vi "ConfigSQLiteSettingDialog.vi"() -> ()   [LabVIEW 2018]
doc: "[Ver 1.00]\nDESCRIPTION\nThis is is the user interface for the config ini data. This can be used as a pattern to apply to all programs to ensure detail is kept out of the code.\n\nERROR HANDLING\nThrow, log error\n\n------------------------------------------------------------------------\n[Ver 1.00]\nSWatts SSDC 07/04/03"
uses:
  System Config Data Manager Parameter.ctl
  Datamanager.ctl
  <vilib>/event_ctls.llb/eventsource.ctl
  ConfigScreen States.ctl
  ConfigCommand.ctl
  Database/SystemdBCommands.ctl
  Error/ErrorCommand.ctl
  StoreCommand.ctl
  <vilib>/Utility/NIReport.llb/NI_report.lvclass
panel:
  in  "Source":T1 items=["LabVIEW UI"=0, "ActiveX"=1, "User Event"=25]
  in  "Save As Button":bool
  in  "Lock Button":bool
  in  "Section":T2
  in  "Table Control":string[][](table)=[["Password"], ["PhysicsLIMs"], ["LIMSSASDBF"], ["a4bld"], ["User"], ["RUN"], ["N:\\LIMS\\Reports\\"], ["C:\\AWE\\Physics LIMS\\HelpFiles\\Help.html"], ["C:\\AWE\\Physics LIMS\\HelpFiles\\PASStaff.html"], ["C:\\AWE\\Physics LIMS\\HelpFiles\\SASWAS.html"], ["C:\\AWE\\Physics LIMS\\HelpFiles\\PASRoutine.html"], ["C:\\AWE\\Physics LIMS\\HelpFiles\\BeHelp.html"], ["C:\\AWE\\Physics LIMS\\HelpFiles\\Building.html"], ["C:\\AWE\\Physics LIMS\\HelpFiles\\PASVisitor.html"], ["C:\\AWE\\Physics LIMS\\HelpFiles\\BeScheduled.html"], ["C:\\AWE\\Physics LIMS\\HelpFiles\\BeUnscheduled.html"], ["C:\\AWE\\Physics LIMS\\HelpFiles\\BeReports.html"], ["C:\\AWE\\Physics LIMS\\HelpFiles\\PASReports.html"], ["C:\\AWE\\Physics LIMS\\HelpFiles\\QA.html"], ["C:\\AWE\\Physics LIMS\\HelpFiles\\Browse.html"], ["C:\\AWE\\Physics LIMS\\HelpFiles\\LEAD.html"], ["C:\\PHYSICSLIMSRB\\"], ["C:/PHYSICSLIMSRB/"], ["C:\\Program Files\\Seagull\\BarTender\\8.0\\BarTend.exe"], ["C:\\AWE\\Physics LIMS\\Documents\\BartenderLabels\\"], ["10"], [""], [""], [""], [""], [""], [""], [""], [""], [""], [""], [""], [""], [""], [""], [""], [""], [""], [""], [""], [""], [""], [""], [""], [""], ["MANUAL VIS PAS RA.btw"], [""], [""], [""], [""], [""], ["A:\\"], ["N:\\LIMS\\IPSIS\\"], ["C:\\AWE\\Physics LIMS\\Documents\\BartenderLabels\\BEWorklist.btw"], ["N:\\LIMS\\BEFILES\\"], ["COM11"], ["0.02001|0.10|0.50|1.0|2.0"], [">0.02<0.1|>=0.1<0.5|>=0.5<1|>=1<2|>=2"], ["0.02001|0.1|0.5|1.0|2.0"], [">0.02<0.1|>=0.1<0.5|>=0.5<1|>=1<2|>=2"], ["C:\\AWE\\Physics LIMS\\Documents\\SAS\\DailyHPR59.btw"], ["SSDCPDF"]]
  in  "SaveButton":bool
  in  "OK":bool
  in  "PrintButton":bool
  in  "SysParameter":T3=enum."RunStatus"
  in  "Version":string(combo)
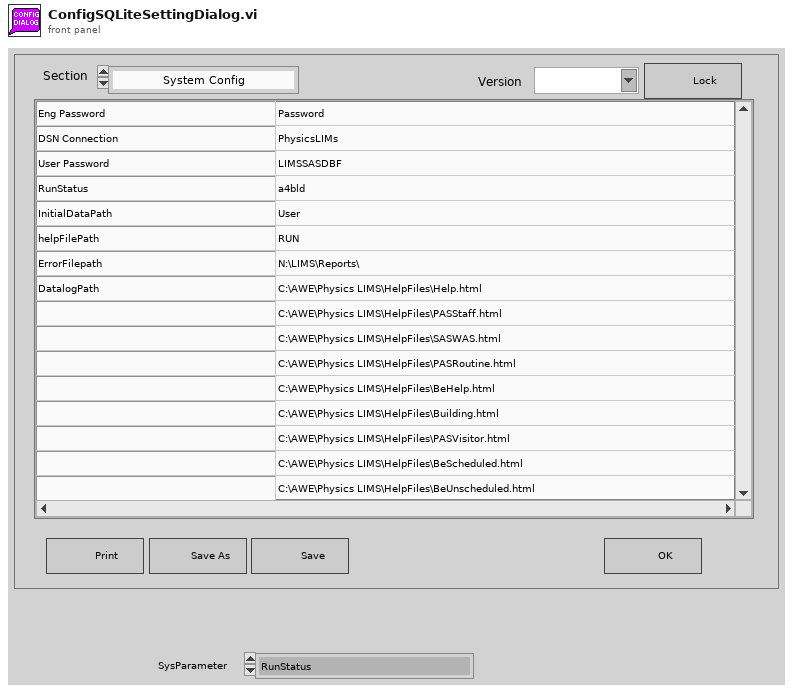
[diagram p1: front panel]
types:
  T1 = typedef "eventsource.ctl" = u32
  T2 = typedef "Datamanager.ctl" = enum16{"System Config"}
  T3 = typedef "System Config Data Manager Parameter.ctl" = enum16{"Eng Password", "DSN Connection", "User Password", "RunStatus", "InitialDataPath", "helpFilePath", "ErrorFilepath", "DatalogPath", "Hello"}
  T4 = typedef "ConfigScreen States.ctl" = enum16{"Initialize", "Run"}
  T5 = typedef "SystemdBCommands.ctl" = enum16{"No Command - Error", "Set Filepath", "Connect dB", "Disconnect dB", "Start Transaction", "Commit", "Rollback", "Describe Table", "Select All From Table", "Fetch Query", "Count Records In Table", "Get User Information", "Get System Config", "Insert New System Config", "UPDATE User Info", "Insert New User", "Get Versions", "Update Key", "Set Version to Default", "Get Default Version", "INSERT Error", "UPDATE Error", "DELETE Errors", "Get All Errors", "Get #Errors for Error"}
  T6 = typedef "ConfigCommand.ctl" = enum16{"No Command - Error", "Initialise Config SQLite", "Save Config", "Get Key", "Set Key", "Update Key", "Get Latest Config Data", "Get Config Data for Version", "Get Default Config Data"}
  T7 = typedef "ErrorCommand.ctl" = enum16{"No Command - Error", "Set to Dev Mode", "Set To Released Mode", "Set Error", "Log Error", "Throw Error", "Log & Throw Error", "Set Error Timed"}
  T8 = typedef "StoreCommand.ctl" = enum16{"No Command - Error", "Store New Version From Inputs", "Update From Input", "Store from dB"}
  T9 = enum16{"Standard Report", "HTML", "Word", "Excel"}
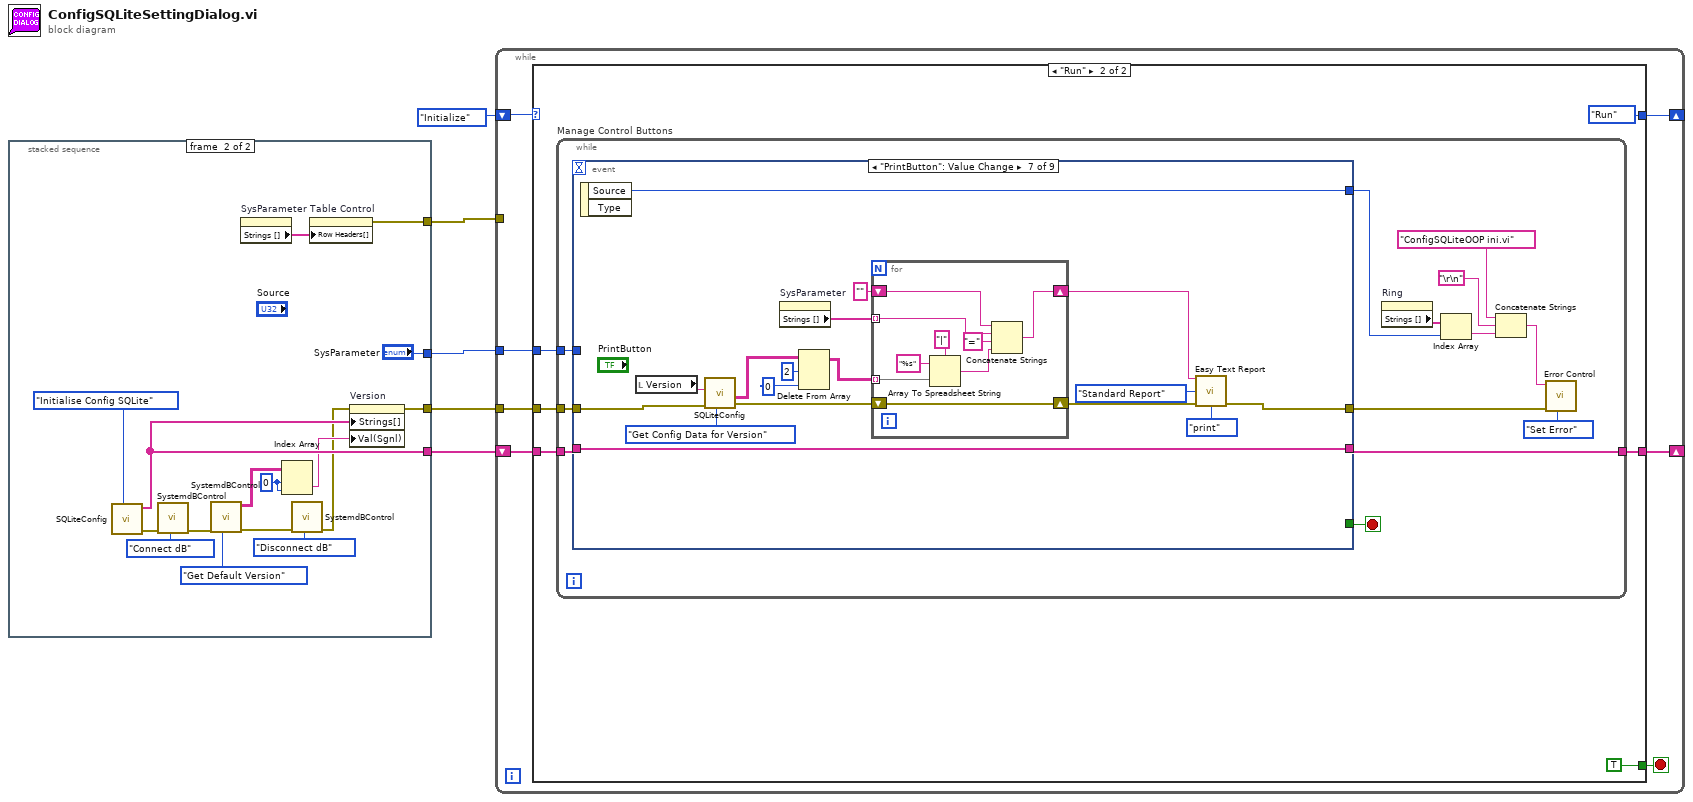
[diagram p0: block diagram]
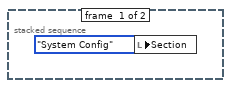
[diagram p2: hidden frame]
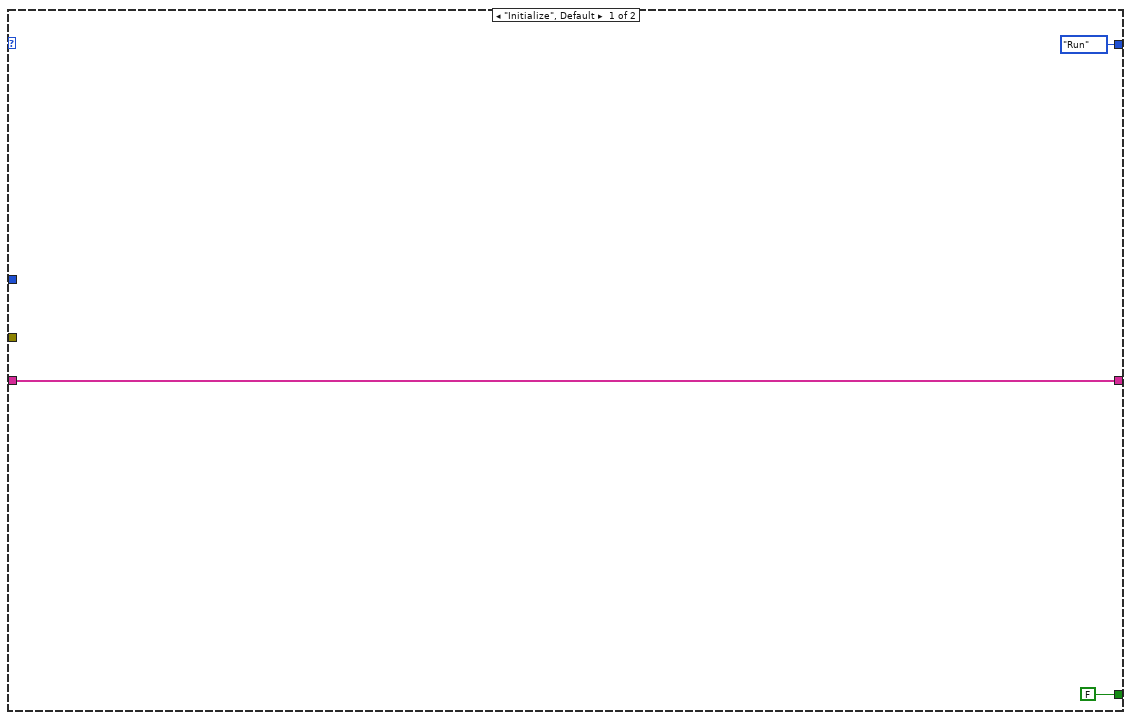
[diagram p3: hidden frame]
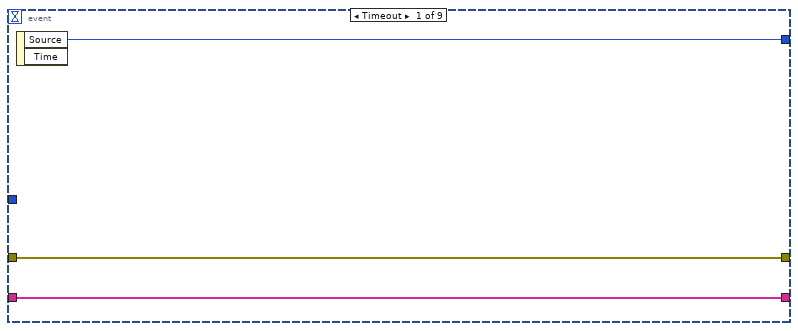
[diagram p4: hidden frame]
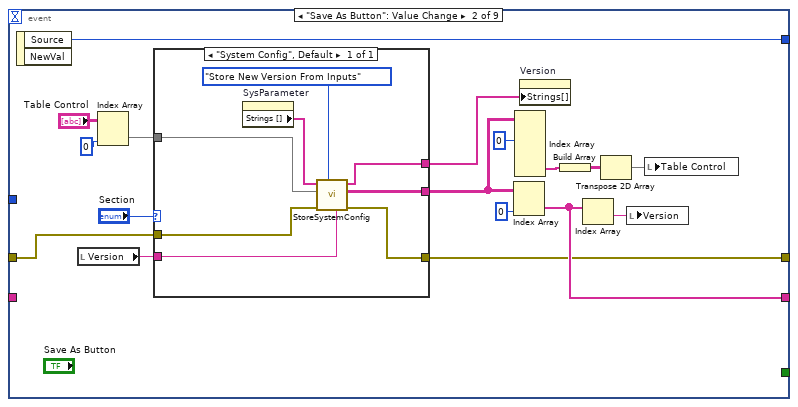
[diagram p5: hidden frame]
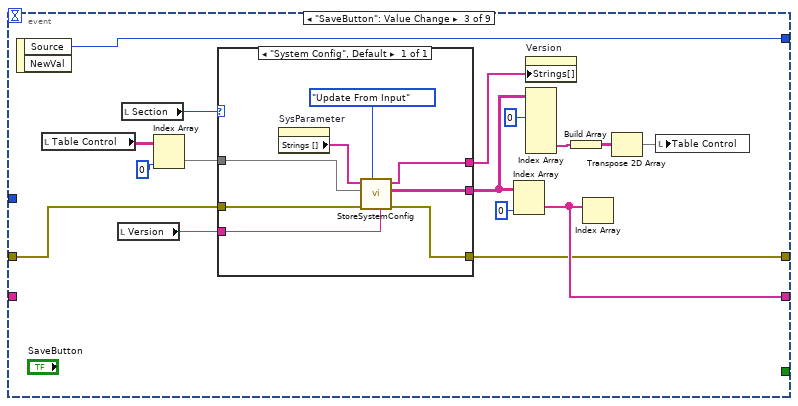
[diagram p6: hidden frame]
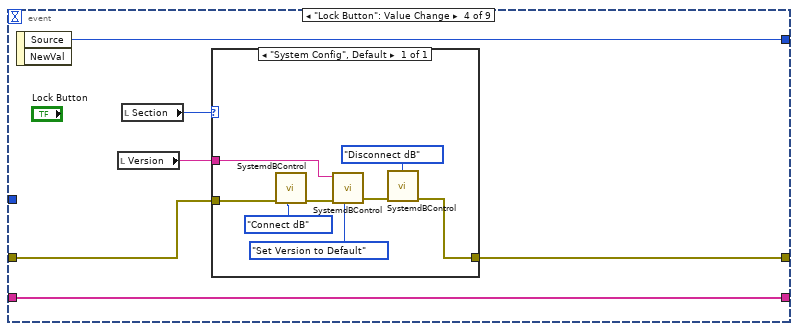
[diagram p7: hidden frame]
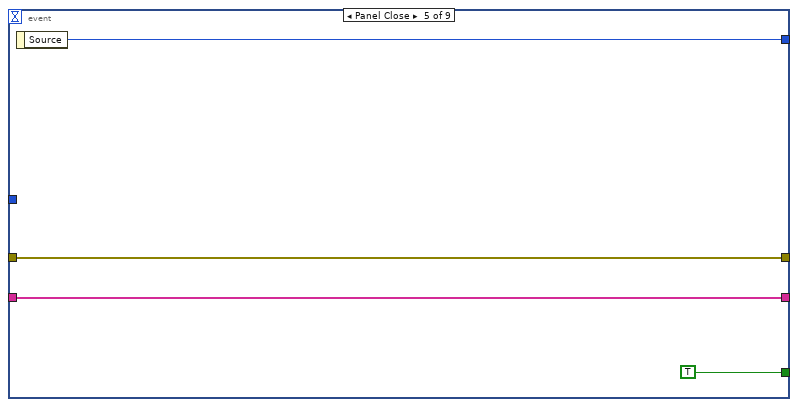
[diagram p8: hidden frame]
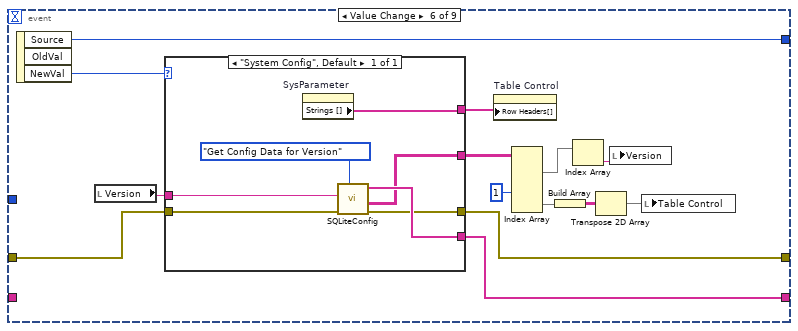
[diagram p9: hidden frame]
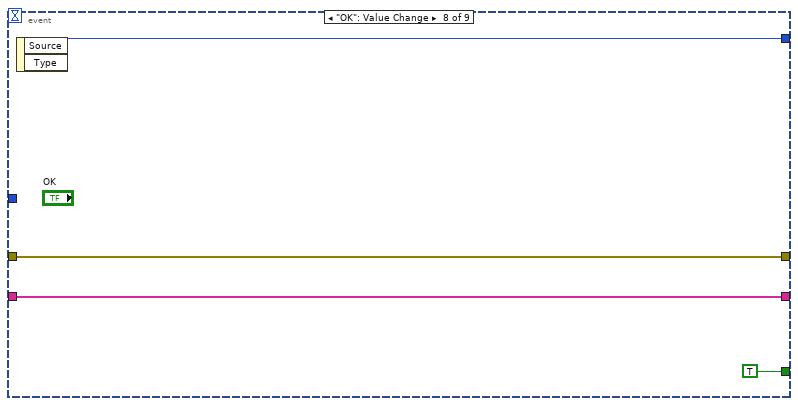
[diagram p10: hidden frame]
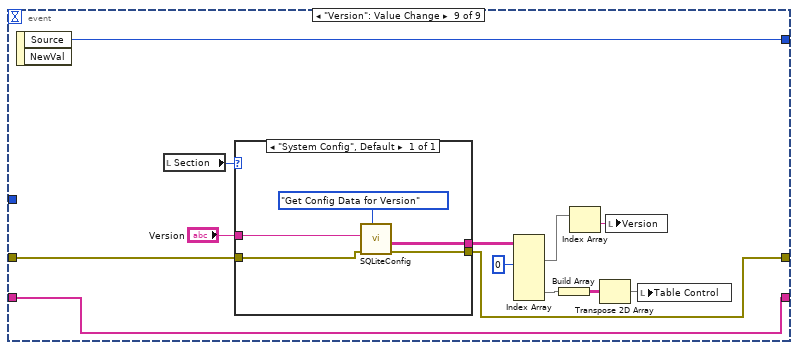
[diagram p11: hidden frame]
diagram:
  n1 = stacked-sequence {
    tunnel: [_ w20] -> w4
    tunnel: [_ "SysParameter"] -> w3
    tunnel: [_ w21] -> w2
    tunnel: [_ w19] -> w1
    frame #0 {
      n2 = local write "Section"(Datamanager."System Config" ("Section")) -> ()
    }
    frame #1 {
      w14 = 0 ("index (row)")
      n3 = call "SQLiteConfig.vi"("ConfigCommand"=ConfigCommand."Initialise Config SQLite") -> ("error out"=w9:errorcluster, "AvailableVersions"=w19:string[])  [unwired: 4 in, 2 out]
      n4 = call "SystemdBControl.vi"("Command"=SystemdBCommands."Connect dB", "error in (no error)"=w9) -> ("error out"=w8:errorcluster)  [unwired: 5 in, 2 out]
      n5 = call "SystemdBControl.vi"("Command"=SystemdBCommands."Get Default Version", "error in (no error)"=w8) -> ("error out"=w11:errorcluster, "Data Out"=w15:string[][])  [unwired: 5 in, 1 out]
      n6 = property on="SysParameter" class="Enum (strict)"() -> ("Strings []"=w18:string[])  [unwired: 2 in, 2 out]
      n7 = Index Array(array=w15, index (row)=w14, index (col)=w14) -> (element=w13:string)
      n8 = call "SystemdBControl.vi"("Command"=SystemdBCommands."Disconnect dB", "error in (no error)"=w11) -> ("error out"=w12:errorcluster)  [unwired: 5 in, 2 out]
      n9 = property on="Table Control" class="Tbl (strict)"("Row Headers[]"=w18) -> (error out=w21:errorcluster)  [unwired: 2 in, 1 out]
      n10 = property on="Version" class="CmbBox"(error in=w12, "Strings[]"=w19, "Val(Sgnl)"=w13) -> (error out=w20:errorcluster)  [unwired: 1 in, 1 out]
    }
  }
  n11 = while {
    shift-right: [w28] -> _
    shift-left: ConfigScreen_States."Initialize" ("Screen State") -> [w29]
    tunnel: w4 -> [w23]
    tunnel: w3 -> [w26]
    tunnel: w2 -> [_]
    shift-right: [w24] -> _
    shift-left: w1 -> [w25]
    stop <- w27 stop-if-true
    n12 = case shown="\"Run\"" w29 {
      tunnel: [ConfigScreen_States."Run" ("Screen State") ConfigScreen_States."Run" ("Screen State")] -> w28
      tunnel: [FALSE TRUE] -> w27
      tunnel: w26 -> [_ w35]
      tunnel: w25 -> [w30 w36]
      tunnel: [w30 w34] -> w24
      tunnel: w23 -> [_ w33]
      frame "Initialize", Default {
      }
      frame "Run" {
        n13 = while "Manage Control Buttons" {
          tunnel: w36 -> [w50]
          tunnel: w35 -> [w49]
          tunnel: [w48] -> w34
          tunnel: w33 -> [w47]
          stop <- w51 stop-if-true
          n14 = event shown="[6] \"PrintButton\": Value Change" {
            selector: _ -> [_ _ _ _ _ _ _ _ _]
            dyn-events: _ -> [_ _ _ _ _ _ _ _ _]
            timeout: _ -> [_ _ _ _ _ _ _ _ _]
            tunnel: [_ _ _ _ TRUE _ _ TRUE _] -> w51
            tunnel: w50 -> [w54 _ _ w107 w120 _ w159 w171 w180]
            tunnel: w49 -> [_ _ _ _ _ _ _ _ _]
            tunnel: [w54 w66 w92 w107 w120 w127 w159 w171 w180] -> w48
            tunnel: w47 -> [w52 w56 w81 w106 w118 w124 w156 w169 w175]
            tunnel: [w52 w55 w80 w104 w118 w123 w149 w169 w174] -> w42
            tunnel: [w53 w57 w82 w105 w119 w122 w148 w170 w173] -> w40
            event Timeout {
              n15 = event-data() -> ("Source"=w53:T1)  [unwired: 1 in, 1 out]
            }
            event "Save As Button": Value Change {
              n16 = event-data() -> ("Source"=w57:T1)  [unwired: 1 in, 1 out]
              n17 = local read "Version"() -> (w58:string)
              n18 = Index Array(array="Table Control", index (col)=0 ("disabled index (col)")) -> (element=w70:string[])  [unwired: 1 in]
              n19 = case shown="\"System Config\", Default" "Section" {
                tunnel: w70 -> [w79]
                tunnel: [w78] -> w60
                tunnel: [w77] -> w62
                tunnel: w58 -> [w74]
                tunnel: w56 -> [w73]
                tunnel: [w72] -> w55
                frame "System Config", Default {
                  n20 = property on="SysParameter" class="Enum (strict)"() -> ("Strings []"=w76:string[])  [unwired: 2 in, 2 out]
                  n21 = call "StoreSystemConfig.vi"("Version"=w74, "StoreConfigCommand"=StoreCommand."Store New Version From Inputs", "error in"=w73, "Table Control"=w79, "Strings []"=w76) -> ("error out"=w72:errorcluster, "All Data"=w78:string[][], "AvailableVersions"=w77:string[])  [unwired: 2 in]
                }
              }
              n22 = Index Array(array=w60, index (col)=0 ("disabled index (col)")) -> (element=w66:string[])  [unwired: 1 in]
              n23 = Index Array(array=w60, index (col) #1=0 ("disabled index (col)")) -> (element #3=w64:string[])  [unwired: 5 in, 2 out]
              n24 = property on="Version" class="CmbBox"("Strings[]"=w62) -> ()  [unwired: 2 in, 2 out]
              n25 = Build Array(w64) -> (w65:string[][])
              n26 = Index Array(array=w66) -> (element=w67:string)  [unwired: 1 in]
              n27 = Transpose 2D Array(2D array=w65) -> (transposed array=w63:string[][])
              n28 = local write "Version"(w67) -> ()
              n29 = local write "Table Control"(w63) -> ()
            }
            event "SaveButton": Value Change {
              n30 = event-data() -> ("Source"=w82:T1)  [unwired: 1 in, 1 out]
              n31 = local read "Table Control"() -> (w84:string[][])
              n32 = local read "Version"() -> (w85:string)
              n33 = local read "Section"() -> (w83:T2)
              n34 = Index Array(array=w84, index (col)=0 ("disabled index (col)")) -> (element=w94:string[])  [unwired: 1 in]
              n35 = case shown="\"System Config\", Default" w83 {
                tunnel: w94 -> [w103]
                tunnel: [w102] -> w87
                tunnel: [w101] -> w88
                tunnel: w85 -> [w98]
                tunnel: w81 -> [w97]
                tunnel: [w96] -> w80
                frame "System Config", Default {
                  n36 = property on="SysParameter" class="Enum (strict)"() -> ("Strings []"=w100:string[])  [unwired: 2 in, 2 out]
                  n37 = call "StoreSystemConfig.vi"("Version"=w98, "StoreConfigCommand"=StoreCommand."Update From Input", "error in"=w97, "Table Control"=w103, "Strings []"=w100) -> ("error out"=w96:errorcluster, "All Data"=w102:string[][], "AvailableVersions"=w101:string[])  [unwired: 2 in]
                }
              }
              n38 = Index Array(array=w87, index (col)=0 ("disabled index (col)")) -> (element=w92:string[])  [unwired: 1 in]
              n39 = property on="Version" class="CmbBox"("Strings[]"=w88) -> ()  [unwired: 2 in, 2 out]
              n40 = Index Array(array=w87, index (col) #1=0 ("disabled index (col)")) -> (element #3=w90:string[])  [unwired: 5 in, 2 out]
              n41 = Build Array(w90) -> (w91:string[][])
              n42 = Index Array(array=w92) -> ()  [unwired: 1 in, 1 out]
              n43 = Transpose 2D Array(2D array=w91) -> (transposed array=w89:string[][])
              n44 = local write "Table Control"(w89) -> ()
            }
            event "Lock Button": Value Change {
              n45 = event-data() -> ("Source"=w105:T1)  [unwired: 1 in, 1 out]
              n46 = local read "Version"() -> (w109:string)
              n47 = local read "Section"() -> (w108:T2)
              n48 = case shown="\"System Config\", Default" w108 {
                tunnel: w109 -> [w112]
                tunnel: w106 -> [w111]
                tunnel: [w110] -> w104
                frame "System Config", Default {
                  n49 = call "SystemdBControl.vi"("Command"=SystemdBCommands."Connect dB", "error in (no error)"=w111) -> ("error out"=w116:errorcluster)  [unwired: 5 in, 2 out]
                  n50 = call "SystemdBControl.vi"("Command"=SystemdBCommands."Set Version to Default", "error in (no error)"=w116, "Data In"=w112) -> ("error out"=w114:errorcluster)  [unwired: 4 in, 2 out]
                  n51 = call "SystemdBControl.vi"("Command"=SystemdBCommands."Disconnect dB", "error in (no error)"=w114) -> ("error out"=w110:errorcluster)  [unwired: 5 in, 2 out]
                }
              }
            }
            event Panel Close {
              n52 = event-data() -> ("Source"=w119:T1)  [unwired: 1 in]
            }
            event Value Change {
              n53 = event-data() -> ("Source"=w122:T1, "NewVal"=w135:T2)  [unwired: 1 in, 1 out]
              n54 = local read "Version"() -> (w126:string)
              n55 = case shown="\"System Config\", Default" w135 {
                tunnel: [w142] -> w134
                tunnel: [w141] -> w127
                tunnel: [w139] -> w125
                tunnel: w126 -> [w140]
                tunnel: w124 -> [w137]
                tunnel: [w136] -> w123
                frame "System Config", Default {
                  n56 = property on="SysParameter" class="Enum (strict)"() -> ("Strings []"=w142:string[])  [unwired: 2 in, 2 out]
                  n57 = call "SQLiteConfig.vi"("ConfigCommand"=ConfigCommand."Get Config Data for Version", "error in (no error)"=w137, "KeyDataIn"=w140) -> ("error out"=w136:errorcluster, "All Data"=w139:string[][], "AvailableVersions"=w141:string[])  [unwired: 2 in, 1 out]
                }
              }
              n58 = property on="Table Control" class="Tbl (strict)"("Row Headers[]"=w134) -> ()  [unwired: 2 in, 2 out]
              n59 = Index Array(array=w125, index (col) #2=1 ("disabled index (col)")) -> (element #1=w133:string[], element #3=w128:string[])  [unwired: 5 in, 1 out]
              n60 = Build Array(w128) -> (w129:string[][])
              n61 = Index Array(array=w133) -> (element=w132:string)  [unwired: 1 in]
              n62 = Transpose 2D Array(2D array=w129) -> (transposed array=w130:string[][])
              n63 = local write "Version"(w132) -> ()
              n64 = local write "Table Control"(w130) -> ()
            }
            event "PrintButton": Value Change {
              n65 = event-data() -> ("Source"=w148:T1)  [unwired: 1 in, 1 out]
              n66 = local read "Version"() -> (w143:string)
              n67 = call "SQLiteConfig.vi"("ConfigCommand"=ConfigCommand."Get Config Data for Version", "error in (no error)"=w156, "KeyDataIn"=w143) -> ("error out"=w153:errorcluster, "All Data"=w147:string[][])  [unwired: 2 in, 2 out]
              n68 = property on="SysParameter" class="Enum (strict)"() -> ("Strings []"=w154:string[])  [unwired: 2 in, 2 out]
              n69 = Delete From Array(array=w147, length=2, index (col)=0 ("disabled index (col)")) -> (array with subset deleted=w144:string[][])  [unwired: 1 in, 1 out]
              n70 = for {
                tunnel: w154 -> [w167] mode=indexing
                shift-right: [w168] -> w152
                shift-left: w153 -> [w168]
                tunnel: w144 -> [w165] mode=indexing
                shift-right: [w160] -> w150
                shift-left: "" ("string") -> [w161]
                n71 = Array To Spreadsheet String(delimiter (Tab)="|", array=w165, 3:"%s" ("format string")) -> (spreadsheet string=w162:string)
                n72 = Concatenate Strings(w161, w167, "=" ("string"), w162) -> (w160:string)
              }
              n73 = call <vilib>:"Easy Text Report.vi"("text to be printed"=w150, "print or save? (Word/Excel/HTML)"=enum16{"print", "save"}."print", "report type (Standard)"=T9."Standard Report" ("report type"), "error in (no error)"=w152) -> ("error out"=w149:errorcluster)  [unwired: 11 in]
            }
            event "OK": Value Change {
              n74 = event-data() -> ("Source"=w170:T1)  [unwired: 1 in, 1 out]
            }
            event "Version": Value Change {
              n75 = event-data() -> ("Source"=w173:T1)  [unwired: 1 in, 1 out]
              n76 = local read "Section"() -> (w179:T2)
              n77 = case shown="\"System Config\", Default" w179 {
                tunnel: "Version" -> [w190]
                tunnel: [w189] -> w177
                tunnel: w175 -> [w187]
                tunnel: [w186] -> w174
                frame "System Config", Default {
                  n78 = call "SQLiteConfig.vi"("ConfigCommand"=ConfigCommand."Get Config Data for Version", "error in (no error)"=w187, "KeyDataIn"=w190) -> ("error out"=w186:errorcluster, "All Data"=w189:string[][])  [unwired: 2 in, 2 out]
                }
              }
              n79 = Index Array(array=w177, index (col) #1=0 ("disabled index (col)")) -> (element #1=w178:string[], element #3=w182:string[])  [unwired: 5 in, 1 out]
              n80 = Build Array(w182) -> (w183:string[][])
              n81 = Index Array(array=w178) -> (element=w184:string)  [unwired: 1 in]
              n82 = Transpose 2D Array(2D array=w183) -> (transposed array=w181:string[][])
              n83 = local write "Version"(w184) -> ()
              n84 = local write "Table Control"(w181) -> ()
            }
          }
          n85 = property on="Ring" class="Ring (strict)"() -> ("Strings []"=w41:string[])  [unwired: 2 in, 2 out]
          n86 = Index Array(array=w41, index=w40) -> (element=w39:string)
          n87 = Concatenate Strings("ConfigSQLiteOOP ini.vi", "\r\n", w39) -> (w44:string)
          n88 = call "Error Control.vi"("Command"=ErrorCommand."Set Error", "error in (no error)"=w42, "Source"=w44) -> ()  [unwired: 5 in, 1 out]
        }
      }
    }
  }
